vi "Weather Station UI.vi"() -> ()   [LabVIEW 2018]
doc: "This is the main VI in the Weather Station Project. It contains the user interface for a temperature warning system. Temperature is retrieved every half second; data is logged when a warning has occurred."
uses:
  Supporting Files/Weather Station States.ctl
  Supporting Files/Weather Data.ctl
  Instance           2 26Saved   Weather Station UI .vi
panel:
  out "Warning":string
  in  "Lower Limit":dbl=20.0
  in  "Upper Limit":dbl=30.0
  in  "Stop Button":bool
  out "Temperature History":dbl(graph)
  # "Temperature Ranges (C)"
  # "Freeze"
  # "Heat \nStroke"
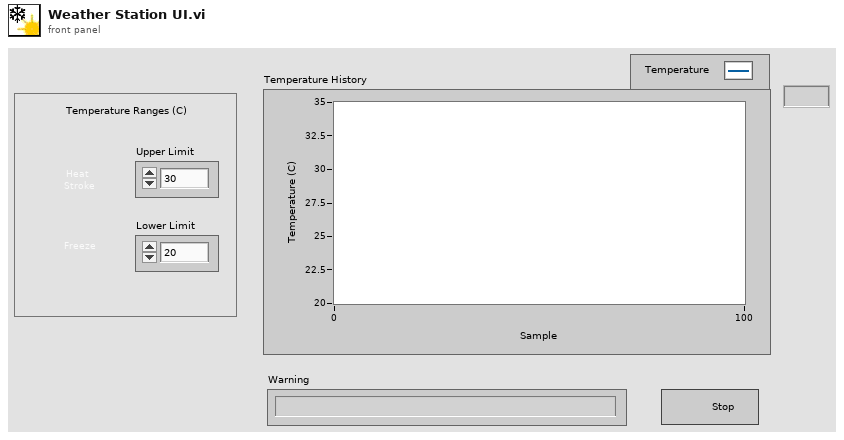
[diagram p1: front panel]
types:
  T1 = enum16{"open", "replace", "create", "open or create", "replace or create", "replace or create with confirmation"}
  T2 = typedef "Weather Data.ctl" = cluster{"Current Temperature":dbl, "Max Temperature":dbl, "Min Temperature":dbl, "Temperature Warning?":bool, "Temperature Warning Text":string}
  T3 = typedef "Weather Station States.ctl" = enum16{"Acquisition", "Range Check", "Analysis", "Data Log", "Time Check"}
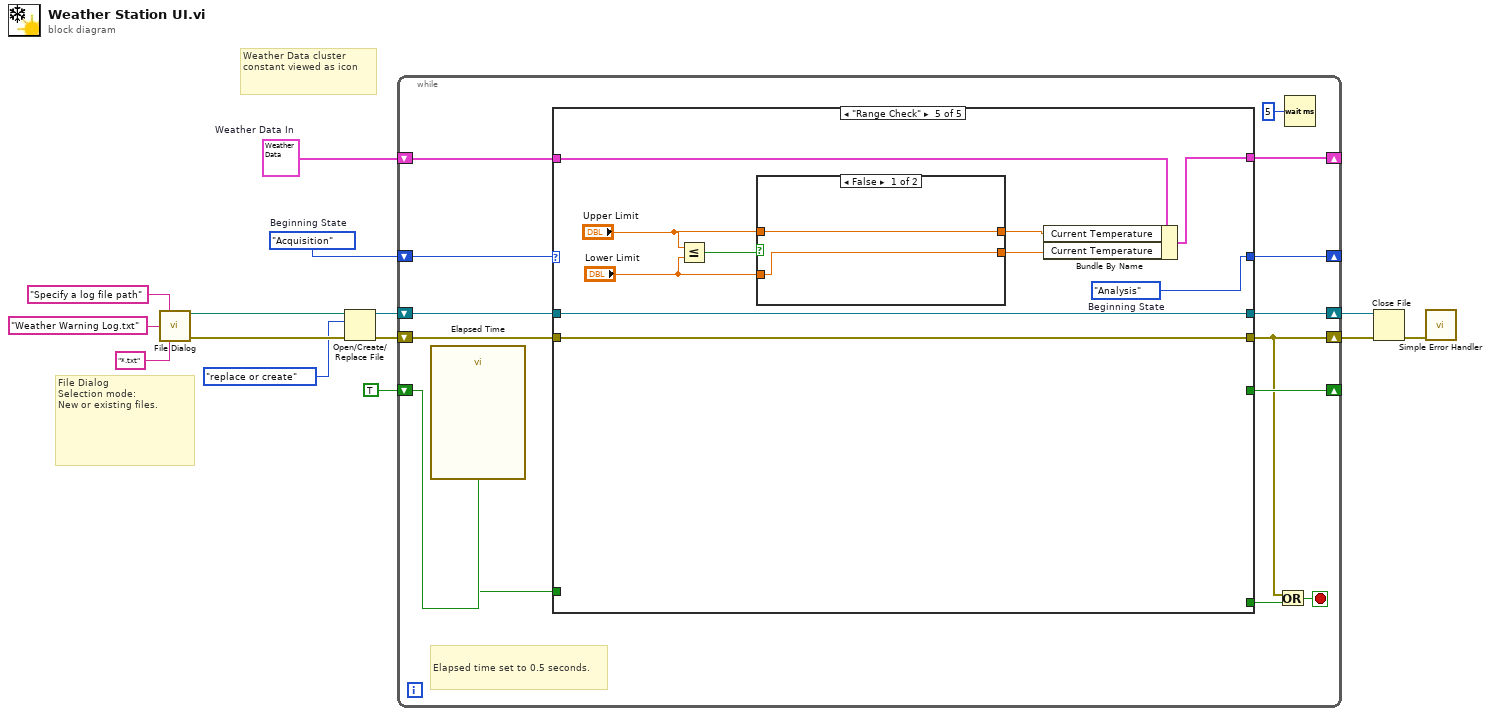
[diagram p0: block diagram]
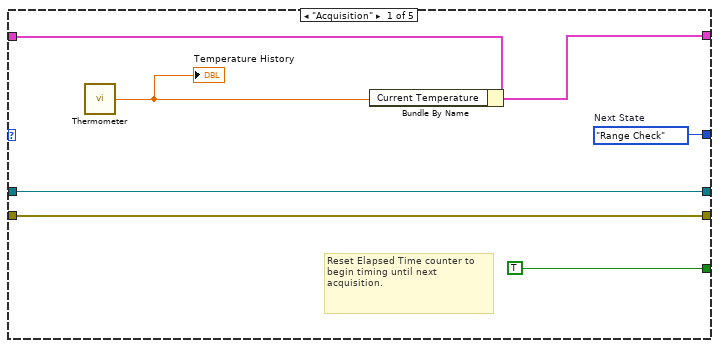
[diagram p2: hidden frame]
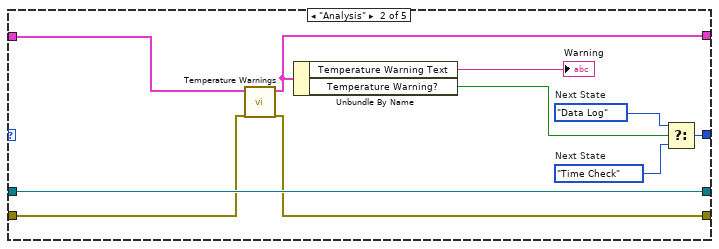
[diagram p3: hidden frame]
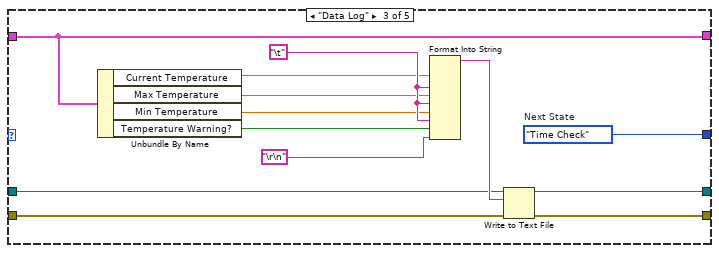
[diagram p4: hidden frame]
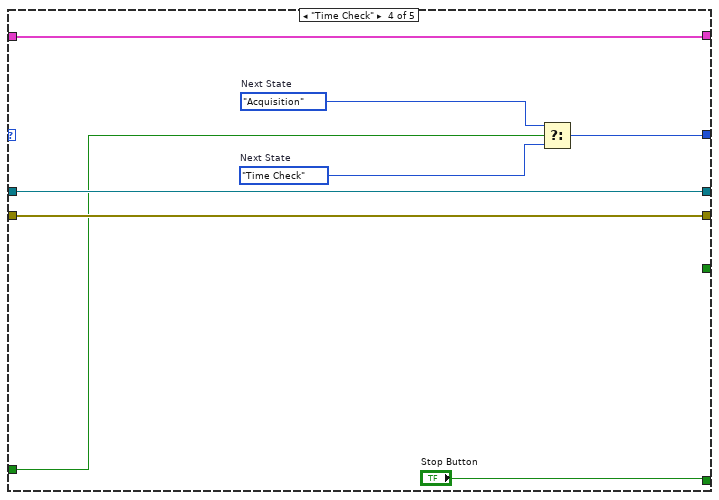
[diagram p5: hidden frame]
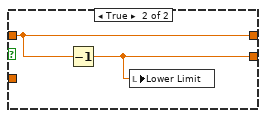
[diagram p6: hidden frame]
diagram:
  w7 = T2 {"Current Temperature"=0.0, "Max Temperature"=0.0, "Min Temperature"=0.0, "Temperature Warning?"=FALSE, "Temperature Warning Text"="No Warning"}  # Weather Data In
  w14 = Weather_Station_States."Acquisition"  # Beginning State
  # "File Dialog\nSelection mode:\nNew or existing files."
  # "Weather Data cluster\nconstant viewed as icon"
  n1 = call "File Dialog"("prompt"="Specify a log file path", "default name"="Weather Warning Log.txt", "pattern (all files)"="*.txt" ("pattern label")) -> ("selected path"=w6:path, "error out"=w3:errorcluster)  [unwired: 9 in, 2 out]
  n2 = Open/Create/Replace File(file path (use dialog)=w6, error in=w3, operation (0:open)=T1."replace or create") -> (refnum out=w9:refnum<file>, error out=w8:errorcluster)  [unwired: 3 in, 1 out]
  n3 = while {
    shift-right: [w27] -> _
    shift-left: w14 -> [w28]
    shift-right: [w15] -> w13
    shift-left: w8 -> [w26]
    shift-right: [w16] -> _
    shift-left: w7 -> [w23]
    shift-right: [w24] -> w12
    shift-left: w9 -> [w22]
    shift-right: [w17] -> _
    shift-left: TRUE ("stop") -> [w19]
    stop <- w25 stop-if-true
    # "Elapsed time set to 0.5 seconds."
    n4 = call "Elapsed Time"("Reset"=w19) -> ("Time has Elapsed"=w18:bool)  [unwired: 11 in, 7 out]
    n5 = case shown="\"Range Check\"" w28 {
      tunnel: [w35 w39 w58 w59 w67] -> w27
      tunnel: [w30 w43 w56 w65 w73] -> w15
      tunnel: w26 -> [w30 w44 w57 w65 w73]
      tunnel: [w34 w45 w55 w66 w72] -> w24
      tunnel: [w31 w38 w46 w64 w68] -> w16
      tunnel: w23 -> [w32 w36 w46 w64 w69]
      tunnel: w22 -> [w34 w45 w53 w66 w72]
      tunnel: [_ _ _ "Stop Button" _] -> w21
      tunnel: w18 -> [_ _ _ w60 _]
      tunnel: [TRUE ("stop") _ _ _ _] -> w17
      frame "Acquisition" {
        w35 = Weather_Station_States."Range Check"  # Next State
        # "Reset Elapsed Time counter to begin timing until next acquisition."
        n6 = call "Thermometer.vi"() -> ("Temperature"=w29:dbl)  [unwired: 1 in]
        "Temperature History" <- w29
        n7 = Bundle By Name(cluster=w32, "Current Temperature"=w29) -> (w31:T2)
      }
      frame "Analysis" {
        w41 = Weather_Station_States."Data Log"  # Next State
        w40 = Weather_Station_States."Time Check"  # Next State
        n8 = call "Temperature Warnings.vi"("Error In"=w44, "Weather Data In"=w36) -> ("Error Out"=w43:errorcluster, "Weather Data Out"=w38:T2)  [unwired: 8 in]
        n9 = Unbundle By Name(w38) -> ("Temperature Warning Text"=→"Warning":string, "Temperature Warning?"=w42:bool)
        n10 = Select(t=w41, s=w42, f=w40) -> (s? t:f=w39:T3)
      }
      frame "Data Log" {
        w58 = Weather_Station_States."Time Check"  # Next State
        w52 = "\t"
        n11 = Unbundle By Name(w46) -> ("Current Temperature"=w51:dbl, "Max Temperature"=w50:dbl, "Min Temperature"=w49:dbl, "Temperature Warning?"=w48:bool)
        n12 = Format Into String(w51, w52, w50, w52, w49, w52, w48, "\r\n") -> (resulting string=w54:string)  [unwired: 3 in, 1 out]
        n13 = Write to Text File(file (use dialog)=w53, text=w54, error in=w57) -> (refnum out=w55:refnum<file>, error out=w56:errorcluster)  [unwired: 1 in, 1 out]
      }
      frame "Time Check" {
        w62 = Weather_Station_States."Time Check"  # Next State
        w61 = Weather_Station_States."Acquisition"  # Next State
        n14 = Select(t=w61, s=w60, f=w62) -> (s? t:f=w59:T3)
      }
      frame "Range Check" {
        w67 = Weather_Station_States."Analysis"  # Beginning State
        n15 = Less Or Equal?(x="Upper Limit", y="Lower Limit") -> (x <= y?=w76:bool)
        n16 = case shown="False" w76 {
          tunnel: "Upper Limit" -> [w78 w80]
          tunnel: "Lower Limit" -> [w77 _]
          tunnel: [w78 w80] -> w71
          tunnel: [w77 w79] -> w70
          frame False {
          }
          frame True {
            n17 = Decrement(x=w80) -> (x-1=w79:dbl)
            n18 = local write "Lower Limit"(w79) -> ()
          }
        }
        n19 = Bundle By Name(cluster=w69, "Current Temperature"=w71, "Current Temperature"=w70) -> (w68:T2)
      }
    }
    n20 = Or(x=w15, y=w21) -> (x .or. y?=w25:bool)
    n21 = Wait (ms)(milliseconds to wait=u32 5 ("y")) -> ()  [unwired: 1 out]
  }
  n22 = Close File(refnum=w12, error in=w13) -> (error out=w11:errorcluster)  [unwired: 1 out]
  n23 = call <vilib>:"Simple Error Handler.vi"("error in (no error)"=w11) -> ()  [unwired: 4 in, 5 out]
